vi "Test Result judgment.vi"(7 "Step Time":timestamp, 9 "=/!=":bool=TRUE, 10 "Return":string, 11 "Limit":string[](array[string])) -> (1 "Step Time":string, 2 "Result":bool, 3 "当前时间":timestamp)   [LabVIEW 2017]
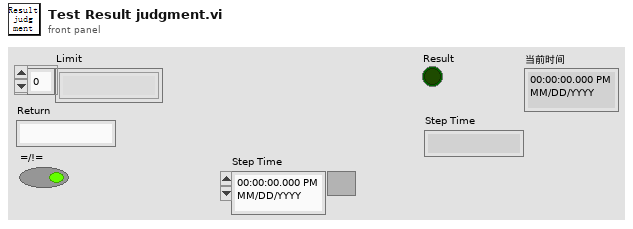
[diagram p1: front panel]
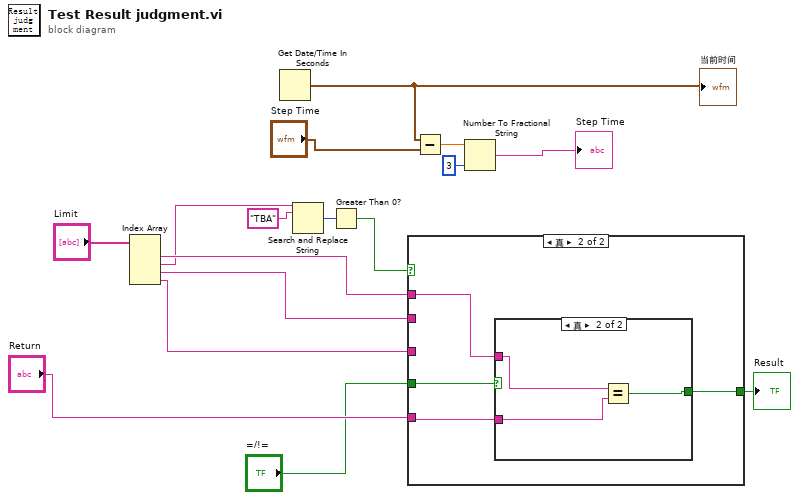
[diagram p0: block diagram]
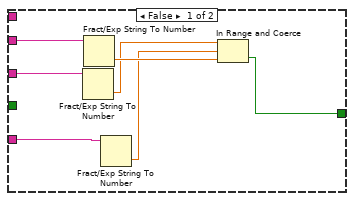
[diagram p2: hidden frame]
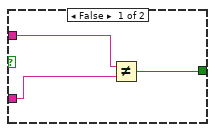
[diagram p3: hidden frame]
diagram:
  n1 = Index Array(array="Limit") -> (element #1=w13:string, element #2=w10:string, element #3=w9:string, element #4=w8:string)  [unwired: 4 in]
  n2 = Get Date/Time In Seconds() -> (seconds since 1Jan1904=w6:timestamp)
  "当前时间" <- w6
  n3 = Search and Replace String(input string=w10, search string="TBA") -> (number of replacements=w15:i32)  [unwired: 6 in, 3 out]
  n4 = Greater Than 0?(x=w15) -> (x > 0?=w14:bool)
  n5 = case shown="真" w14 {
    tunnel: w13 -> [_ w26]
    tunnel: [w17 w27] -> w7
    tunnel: "Return" -> [w23 w25]
    tunnel: w9 -> [w22 _]
    tunnel: w8 -> [w21 _]
    tunnel: "=/!=" -> [_ w24]
    frame False {
      n6 = Fract/Exp String To Number(string=w21) -> (number=w19:dbl)  [unwired: 3 in, 1 out]
      n7 = Fract/Exp String To Number(string=w22) -> (number=w20:dbl)  [unwired: 3 in, 1 out]
      n8 = Fract/Exp String To Number(string=w23) -> (number=w18:dbl)  [unwired: 3 in, 1 out]
      n9 = In Range and Coerce(upper limit=w19, x=w18, lower limit=w20) -> (In Range?=w17:bool)  [unwired: 1 out]
    }
    frame True {
      n10 = case shown="真" w24 {
        tunnel: [w28 w33] -> w27
        tunnel: w26 -> [w30 w32]
        tunnel: w25 -> [w29 w31]
        frame False {
          n11 = Not Equal?(x=w30, y=w29) -> (x != y?=w28:bool)
        }
        frame True {
          n12 = Equal?(x=w32, y=w31) -> (x = y?=w33:bool)
        }
      }
    }
  }
  "Result" <- w7
  n13 = Subtract(x=w6, y="Step Time") -> (x-y=w4:dbl)
  n14 = Number To Fractional String(number=w4, precision (6)=i16 3 ("精度(6)")) -> (F-format string=→"Step Time":string)  [unwired: 2 in]
